vi "MDAQ_GetTimeTemp.vi"(4 "Elapsed Time Ref":refnum<vi>, 7 "Delta T (s) Ref":refnum<vi>, 8 "State in":T4=enum."ClearCVCycle", 9 "Cluster In":T2 {"CV"."Temperature Array" scale=0.0..100.0}, 10 "Status In":T1 {"GATESTOP" format="%04x"; "GATESTRT" format="%04x"; "AMPLITUDE" format="%04x"; "M_CYCLES" format="%04x"; "N_CYCLES" format="%04x"; "STEP" format="%04x"; "BASE" format="%04x"; "CHAN" format="%04x"}, 11 "CV-Prog Ref":refnum<vi>) -> (0 "State Out":T4=enum."ClearCVCycle", 1 "Cluster Out":T2 {"CV"."Temperature Array" scale=0.0..100.0}, 2 "Status Out":T1 {"GATESTOP" format="%04x"; "GATESTRT" format="%04x"; "AMPLITUDE" format="%04x"; "M_CYCLES" format="%04x"; "N_CYCLES" format="%04x"; "STEP" format="%04x"; "BASE" format="%04x"; "CHAN" format="%04x"}, 6 "Temps":cluster{"Double":dbl, "Double":dbl})   [LabVIEW 2021]
uses:
  Status_Def.ctl
  GUI_Def.ctl
  Mode_Enum.ctl
  Status_Cluster.ctl
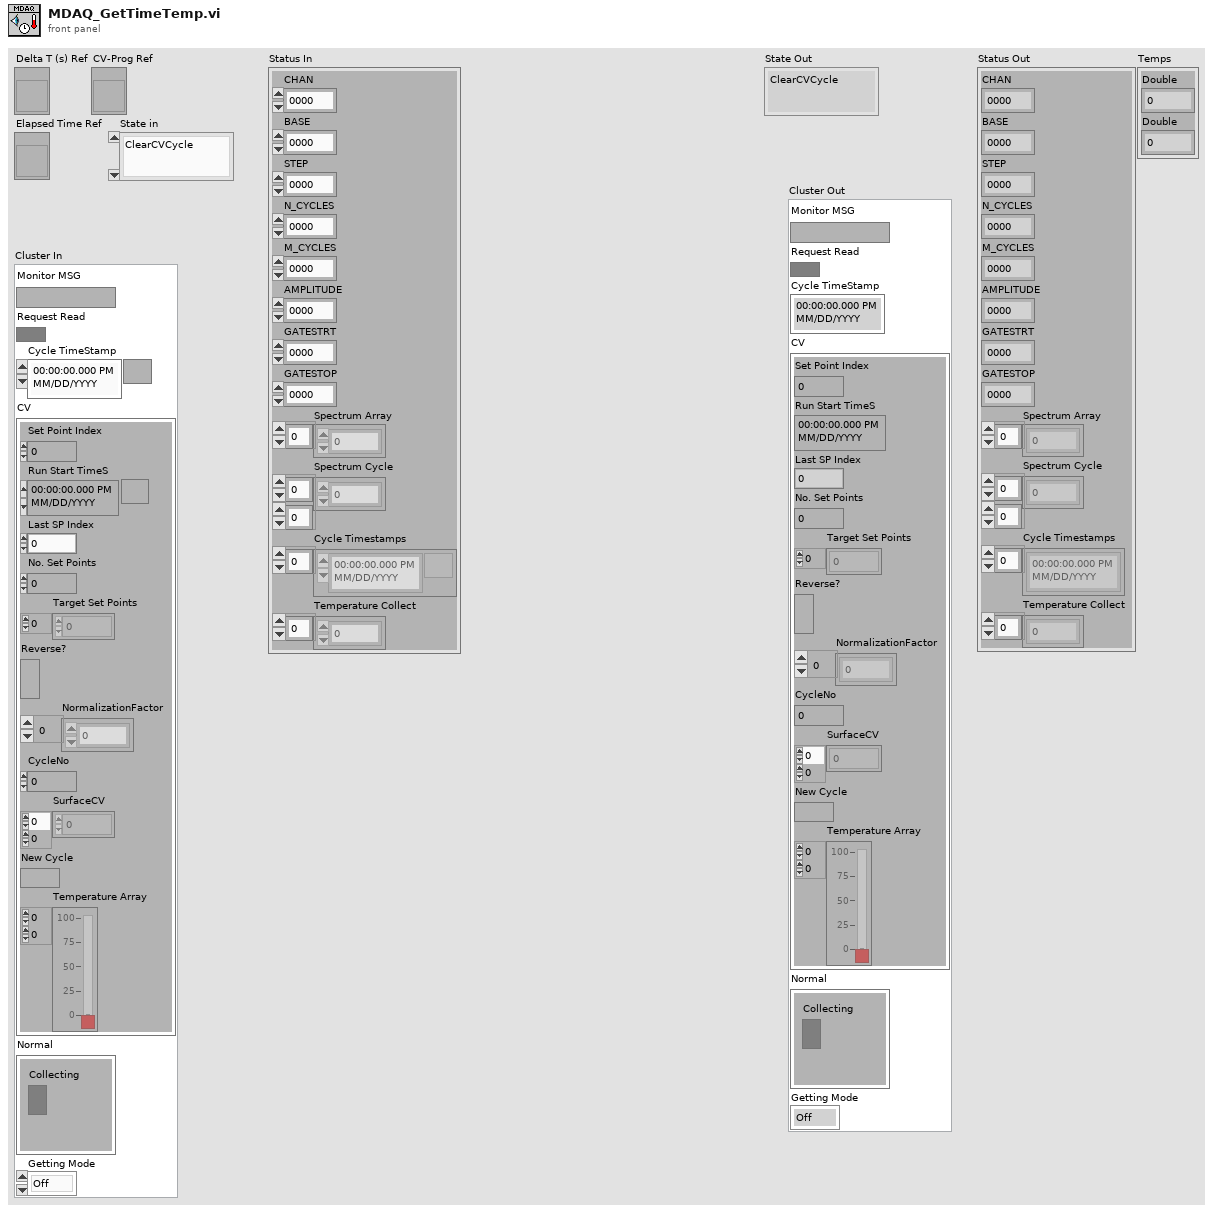
[diagram p1: front panel]
types:
  T1 = typedef "Status_Cluster.ctl" = cluster{"CHAN":u32, "BASE":u32, "STEP":u32, "N_CYCLES":u32, "M_CYCLES":u32, "AMPLITUDE":u32, "GATESTRT":u32, "GATESTOP":u32, "Spectrum Array":u32[], "Spectrum Cycle":u32[][], "Cycle Timestamps":timestamp[], "Temperature Collect":dbl[]}
  T2 = typedef "GUI_Def.ctl" = cluster{"Monitor MSG":string, "Request Read":bool, "Cycle TimeStamp":timestamp, "CV":cluster{"Set Point Index":u32, "Run Start TimeS":timestamp, "Last SP Index":u32, "No. Set Points":u32, "Target Set Points":i32[], "Reverse?":bool, "NormalizationFactor":i32[], "CycleNo":i32, "SurfaceCV":dbl[][], "New Cycle":bool, "Temperature Array":dbl[][]}, "Normal":cluster{"Collecting":bool}, "Getting Mode":T3}
  T3 = typedef "Mode_Enum.ctl" = enum16{"Off", "Normal", "CV+Temp", "CV"}
  T4 = typedef "Status_Def.ctl" = enum16{"ConfigCVCycle", "ClearCVCycle", "WriteCVData", "SendRamp", "LoadSpectrum", "RefreshCV", "SaveCVPlot", "GetCVSpectrum", "ConfigCV", "StopCV", "StartCV", "SaveSpectrum", "Clear Spectrum", "StopCollecting", "StopAq", "StartAq", "Reset MDAQ", "Get Spectrum", "Clear Monitor", "Idle", "String Send", "Settings Send", "Read Help"}
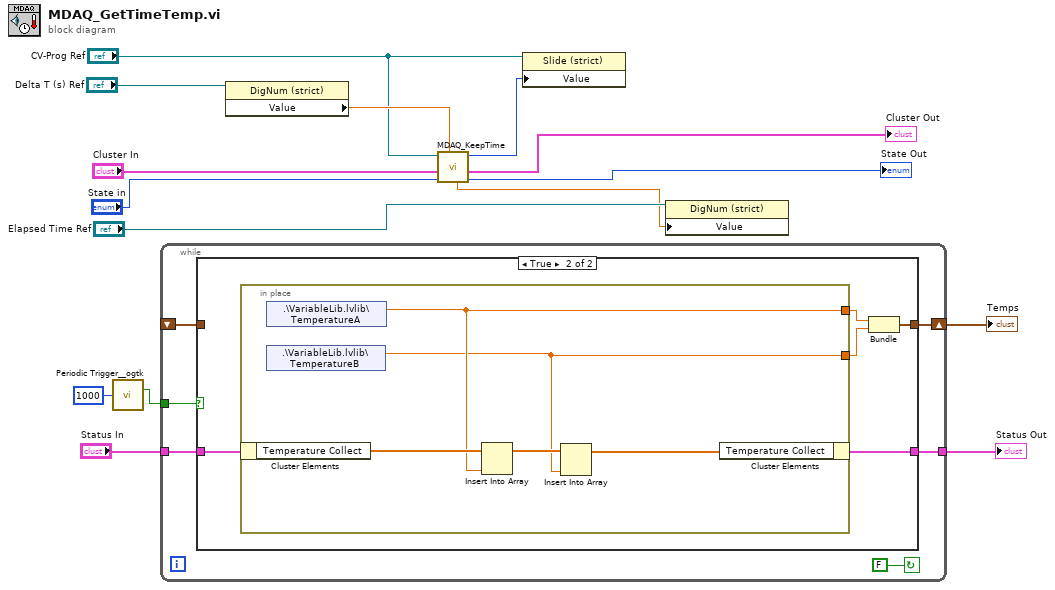
[diagram p0: block diagram]
diagram:
  n1 = call <userlib>:"Periodic Trigger__ogtk.vi"("time (ms)"=u32 1000) -> ("Triggered"=w2:bool)  [unwired: 12 in, 2 out]
  n2 = while {
    tunnel: w2 -> [w18]
    shift-right: [w19] -> w3
    shift-left: _ -> [w16]
    tunnel: "Status In" -> [w21]
    tunnel: [w20] -> w4
    stop <- FALSE continue-if-true
    n3 = case shown="True" w18 {
      tunnel: w21 -> [w23 w28]
      tunnel: [w23 w27] -> w20
      tunnel: [w22 w24] -> w19
      tunnel: w16 -> [w22 _]
      frame False {
      }
      frame True {
        n4 = in-place {
          in-place-border: [w30] -> w26
          in-place-border: [w29] -> w25
          n5 = in-place-cluster #1(w28) -> ("Temperature Collect"=w33:dbl[])
          n6 = shared-variable ".\\VariableLib.lvlib\\TemperatureA"() -> (w30:dbl)  [unwired: 1 in, 1 out]
          n7 = shared-variable ".\\VariableLib.lvlib\\TemperatureB"() -> (w29:dbl)  [unwired: 1 in, 1 out]
          n8 = Insert Into Array(array=w33, new element=w30) -> (w32:dbl[])  [unwired: 1 in]
          n9 = Insert Into Array(array=w32, new element=w29) -> (w31:dbl[])  [unwired: 1 in]
          n10 = in-place-cluster #1("Temperature Collect"=w31) -> (w27:T1)
        }
        n11 = Bundle("Double"=w26, "Double"=w25) -> (w24:cluster{"Double":dbl, "Double":dbl})  [unwired: 1 in]
      }
    }
  }
  "Status Out" <- w4
  "Temps" <- w3
  n12 = property class="DigNum (strict)"(reference="Delta T (s) Ref") -> ("Value"=w14:dbl)  [unwired: 1 in, 2 out]
  n13 = call "MDAQ_KeepTime.vi"("Delta T (s)"=w14, "State in"="State in", "Cluster In"="Cluster In", "Slide in"="CV-Prog Ref") -> ("State Out"=→"State Out":T4, "Cluster Out"=→"Cluster Out":T2, "Progress"=w13:u8, "Elapsed Out"=w10:dbl)  [unwired: 4 in]
  n14 = property class="Slide (strict)"(reference="CV-Prog Ref", "Value"=w13) -> ()  [unwired: 1 in, 2 out]
  n15 = property class="DigNum (strict)"(reference="Elapsed Time Ref", "Value"=w10) -> ()  [unwired: 1 in, 2 out]
